vi "switchToAdmin.vi"(8 "error in (no error)":errorcluster, 11 "SystemSettings in":refnum<class "SystemSettings.lvclass">) -> (0 "error out":errorcluster, 3 "SystemSettings out":refnum<class "SystemSettings.lvclass">)   [LabVIEW 2016, in "SystemSettings.lvclass"]
uses:
  SystemSettings.lvclass
panel:
  out "return code":i32
  out "standard error":string
  out "standard output":string
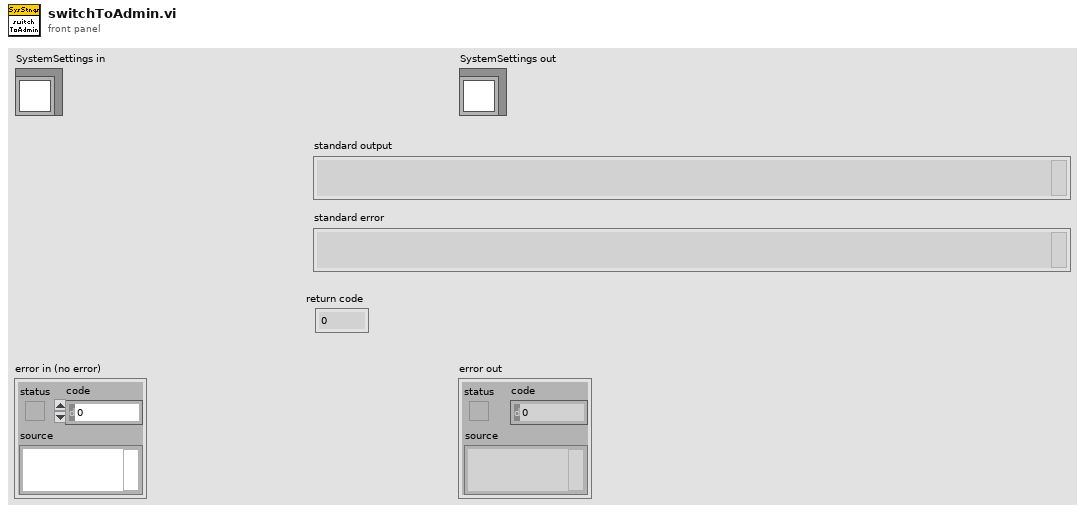
[diagram p1: front panel]
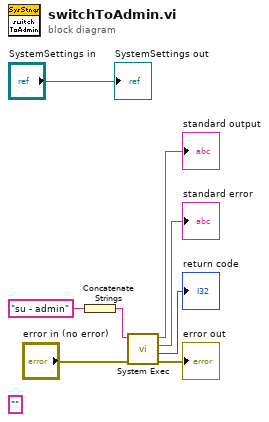
[diagram p0: block diagram]
diagram:
  (unwired) "" ("string")
  n1 = Concatenate Strings("su - admin" ("string")) -> (w7:string)
  n2 = call <vilib>:"System Exec.vi"("error in (no error)"="error in (no error)", "command line"=w7) -> ("error out"=→"error out":errorcluster, "return code"=→"return code":i32, "standard error"=→"standard error":string, "standard output"=→"standard output":string)  [unwired: 6 in]
  "SystemSettings out" <- "SystemSettings in"
